vi "buzzer activo y passivo.vi"() -> ()   [LabVIEW 2016]
uses:
  <vilib>/LabVIEW Interface for Arduino/Type Defs/Board Type.ctl
  <vilib>/LabVIEW Interface for Arduino/Type Defs/Connection Type.ctl
  <vilib>/LabVIEW Interface for Arduino/LabVIEW Interface for Arduino.lvlib
panel:
  in  "stop":bool
  in  "Pasivo":u32(knob) scale=0.0..1000.0
  in  "Activo":u32(knob) scale=0.0..255.0
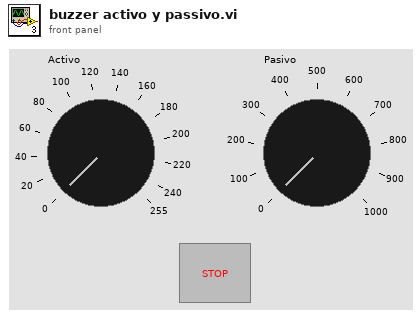
[diagram p1: front panel]
types:
  T1 = typedef "LabVIEW Interface for Arduino.lvlib/Connection Type.ctl" = enum8{"USB / Serial", "XBEE", "BlueSmirf (Bluetooth)"}
  T2 = typedef "LabVIEW Interface for Arduino.lvlib/Board Type.ctl" = enum16{"Uno", "Dimuelanove w/Atmega 328", "Mega 2560"}
  T3 = typedef "LabVIEW Interface for Arduino.lvlib/Arduino Resource.ctl" = cluster{"VISA resource":refnum<visa-resource-name>, "Board Type":T2, "Connection Type":enum8{"USB / Serial"}, "Bytes Per Packet (15)":u8}
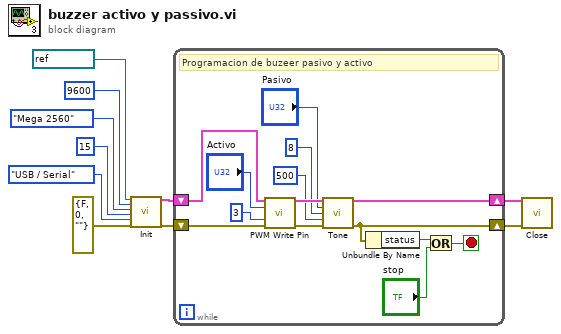
[diagram p0: block diagram]
diagram:
  n1 = call <vilib>:"Init.vi"("VISA resource"=refnum<visa-resource-name> "COM6", "Baud Rate (115200)"=u32 9600, "Board Type (Uno)"=Board_Type."Mega 2560", "Bytes Per Packet (15)"=u32 15, "Connection Type (USB/Serial)"=Connection_Type."USB / Serial", "error in"=errorcluster {"status"=FALSE, "code"=0, "source"=""}) -> ("Arduino Resource"=w4:T3, "error out"=w3:errorcluster)  [unwired: 12 in]
  n2 = while {
    shift-right: [w11] -> w1
    shift-left: w4 -> [w24]
    shift-right: [w12] -> w2
    shift-left: w3 -> [w23]
    stop <- w13 stop-if-true
    # "Programacion de buzeer pasivo y activo"
    n3 = call <vilib>:"PWM Write Pin.vi"("Arduino Resource"=w24, "Duty Cycle (0 - 255)"="Activo", "PWM Pin (3)"=u8 3, "error in"=w23) -> ("Arduino Resource"=w20:T3, "error out"=w19:errorcluster)  [unwired: 10 in]
    n4 = call <vilib>:"Tone.vi"("Arduino Resource"=w20, "Tone DO Pin"="Pasivo", "Frequency (0 Hz)"=u16 8, "Duration (1 ms)"=u32 500, "error in"=w19) -> ("Arduino Resource"=w11:T3, "error out"=w12:errorcluster)  [unwired: 9 in]
    n5 = Unbundle By Name(w12) -> ("status"=w14:bool)
    n6 = Or(x=w14, y="stop") -> (x .or. y?=w13:bool)
  }
  n7 = call <vilib>:"Close.vi"("Arduino Resource"=w1, "error in"=w2) -> ()  [unwired: 13 in, 1 out]
